vi "LIDAR Sensor Fusion.vi"() -> ()   [LabVIEW 2019]
panel:
  in  "Pointed at Target":bool
  out "Fused Range (in)":dbl
  in  "Estimate Range (in)":dbl
  in  "LIDAR Range (in)":dbl
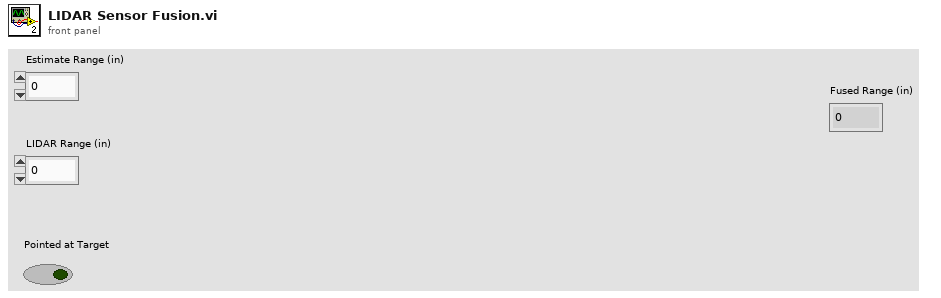
[diagram p1: front panel]
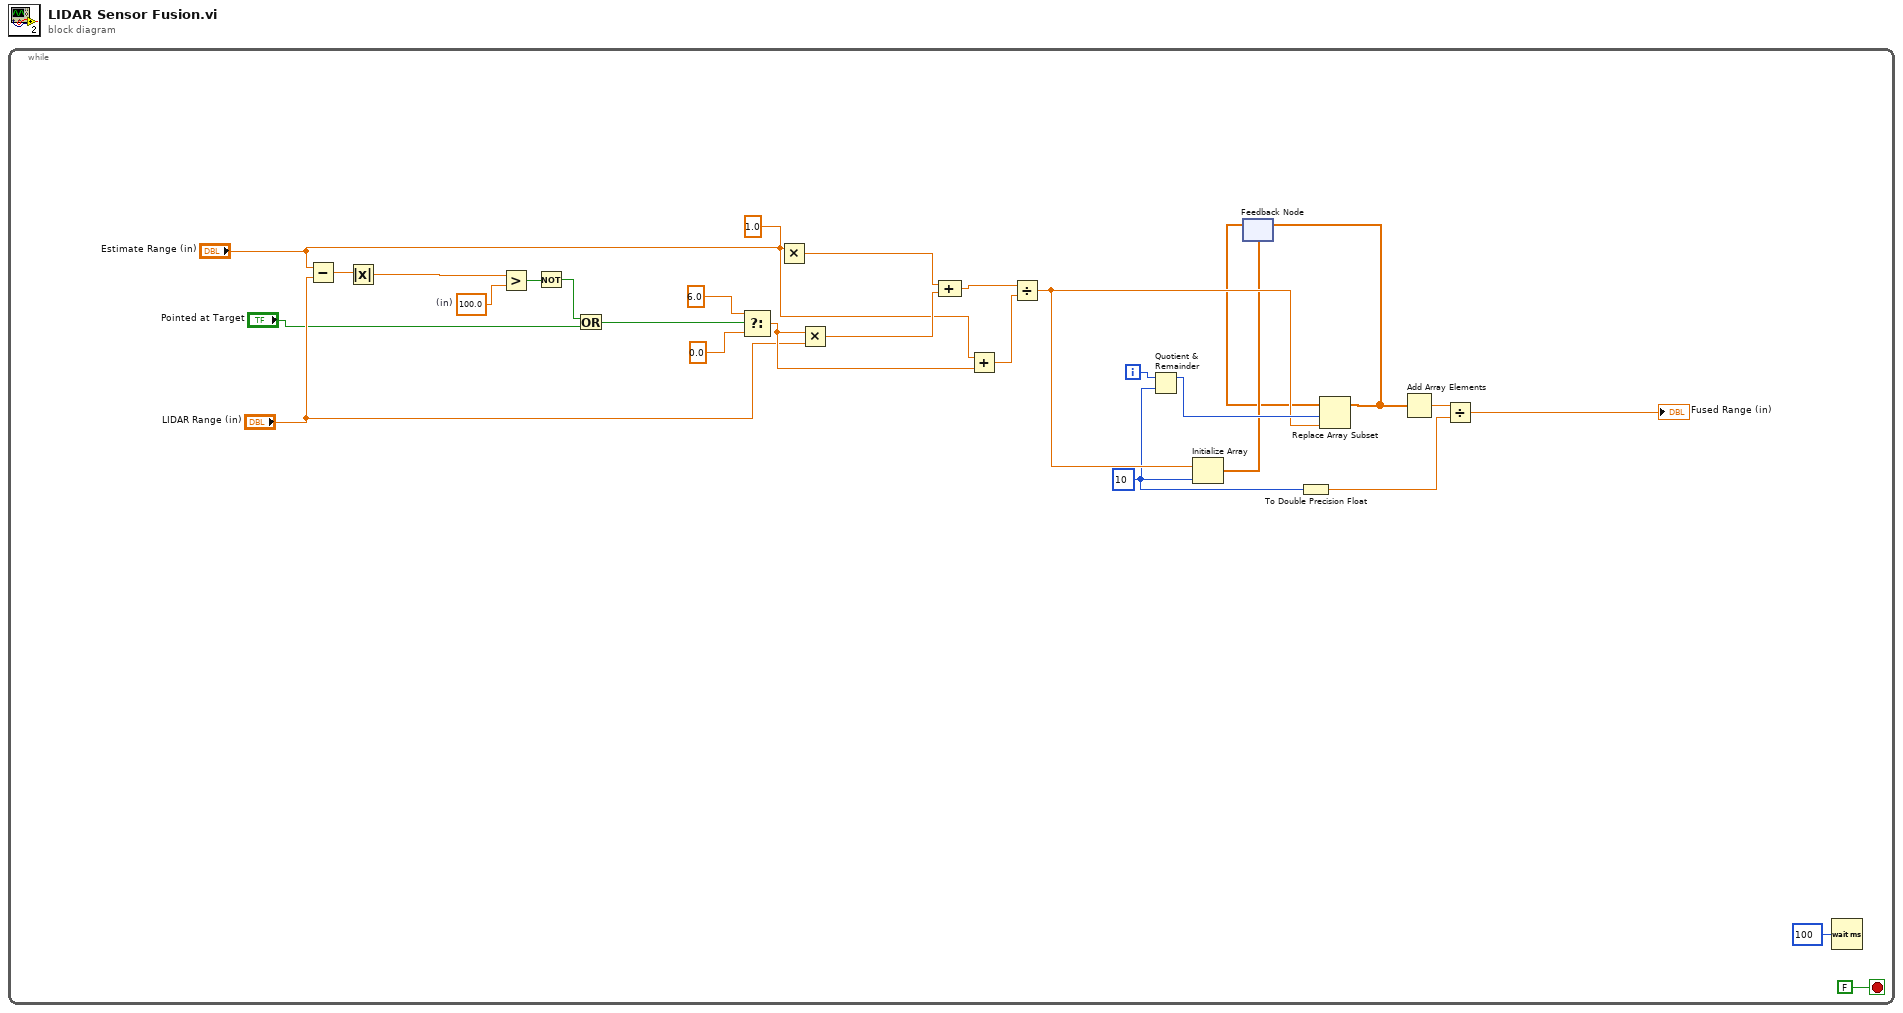
[diagram p0: block diagram]
diagram:
  n1 = while {
    i -> [w10]
    stop <- FALSE stop-if-true
    w6 = 10 ("dimension size")
    w17 = 100.0  # (in)
    w26 = 1.0 ("x")
    n2 = Subtract(x="Estimate Range (in)", y="LIDAR Range (in)") -> (x-y=w19:dbl)
    n3 = Absolute Value(x=w19) -> (abs(x)=w18:dbl)
    n4 = Greater?(x=w18, y=w17) -> (0:w16:bool)
    n5 = Not(x=w16) -> (.not. x?=w15:bool)
    n6 = Or(x=w15, y="Pointed at Target") -> (x .or. y?=w13:bool)
    n7 = Select(t=6.0 ("x"), s=w13, f=0.0) -> (s? t:f=w23:dbl)
    n8 = Multiply(x=w26, y="Estimate Range (in)") -> (x*y=w28:dbl)
    n9 = Multiply(x=w23, y="LIDAR Range (in)") -> (x*y=w27:dbl)
    n10 = Compound Arithmetic op=ADD(w28, w27) -> (w29:dbl)
    n11 = Add(x=w26, y=w23) -> (x+y=w25:dbl)
    n12 = Divide(x=w29, y=w25) -> (x/y=w8:dbl)
    n13 = Quotient & Remainder(x=w10, y=w6) -> (x-y*floor(x/y)=w9:i32)  [unwired: 1 out]
    n14 = Initialize Array(w8, w6) -> (w3:dbl[])
    n15 = feedback #1(w3) -> (w2:dbl[])
    n16 = To Double Precision Float(number=w6) -> (double precision float=w4:dbl)
    n17 = Replace Array Subset(array=w2, new element=w8, index=w9) -> (w1:dbl[])
    n18 = feedback-in #1(w1) -> ()
    n19 = Add Array Elements(numeric array=w1) -> (sum=w7:dbl)
    n20 = Divide(x=w7, y=w4) -> (x/y=→"Fused Range (in)":dbl)
    n21 = Wait (ms)(milliseconds to wait=u32 100) -> ()  [unwired: 1 out]
  }
